vi "Main.vi"() -> ()   [LabVIEW 2015]
doc: "This Continuous Measurement sample project is based on the Queued Message Handler template.\n\nThe Event Handling Loop generates messages based on user interface actions.\n\nThe Message Handling Loop processes messages generated by the Event Handling Loop, or by other messages. There are also Acquisition and Logging message handling loop subVIs, and a chart updating loop."
uses:
  controls/UI Data.ctl
  controls/UI State.ctl
  Acquisition/Generic data packet.ctl
  My Graphs/Gps Map Graph coordinates.ctl
  Settings/Settings.ctl
  Acquisition/Hardware Configuration.ctl
  Logging/Logging Configuration.ctl
  My Graphs/Gps Map Graph config.ctl
  My Graphs/Chart to Graph enum.ctl
  Telemetria_Rotterdam_API_v2/TypeDef/data_graph.ctl
  My Graphs/Gps Map Graph enum.ctl
  Support VIs/Message Queue/Enqueue Message (Single).vi
  Support VIs/Message Queue/Enqueue Message (Array).vi
  <vilib>/Utility/error.llb/Error Cluster From Error Code.vi
  <vilib>/ErrorRing/Error Ring.xnode
  Acquisition/Acquisition.lvlib
  Logging/Logging.lvlib
  Settings/Settings.lvlib
  Support VIs/User Event - Stop/User Event - Stop.lvlib
  Support VIs/Message Queue/Message Queue.lvlib
  My Graphs/My Graphs.lvlib
panel:
  out "RX":bool
  out "EM_RPM_top":u16 caption="EM RPM"
  out "ICE_RPM_top":u16 caption="ICE RPM"
  out "Battery_voltage_top":sgl caption="Battery voltage"
  in  "Disconnect":bool
  out "Status":string
  in  "Exit_top":bool caption="Exit"
  out "Strategy_top":u8 caption="Strategy"
  out "ElettricMotor_top":bool caption="Electric\nMotor"
  out "Electronics_top":bool caption="Electronics"
  out "Emergency_top":bool caption="Emergency"
  out "Humidity2_top":sgl caption="Humidity 2"
  out "Humidity1_top":sgl caption="Humidity 1"
  out "Temperature3_top":sgl caption="Temperature 3"
  out "Temperature2_top":sgl caption="Temperature 2"
  out "Temperature1_top":sgl caption="Temperature 1" format="%_2f"
  out "Speed_top":sgl caption="Speed" format="%_3g"
  out "Current_top":sgl caption="Current" format="%_3f"
  out "Voltage_top":sgl caption="Voltage" format="%_4f"
  in  "Connect":bool
  in  "Tab Control":T1(tab)
  out "TimeRT":string caption="Time"
  out "Humidity 2":sgl(slide) scale=0.0..100.0
  out "Humidity 1":sgl(slide) scale=0.0..100.0
  out "Current":sgl(knob) scale=0.0..10.0
  out "Voltage":sgl(knob) scale=0.0..50.0
  out "Temperature 3":sgl(slide) scale=0.0..100.0
  out "Temperature 2":sgl(slide) scale=0.0..100.0
  out "Temperature 1":sgl(slide) scale=0.0..100.0
  out "Speed":sgl(knob) scale=0.0..40.0
  out "Map":cluster{"X":dbl, "Y":dbl}[](graph)
  out "Electric Motor RPM":u16(knob) scale=0.0..10000.0
  out "ICE RPM":u16(knob) scale=0.0..10000.0
  out "Battery voltage":sgl(knob) scale=0.0..50.0
  out "TimeM":string caption="Time"
  out "Mini Map":cluster{"X":dbl, "Y":dbl}[](graph)
  out "Voltage_Graph":cluster{"Tempi":dbl[], "Valori":dbl[]}[](graph) caption="Voltage"
  out "Current_Graph":cluster{"Tempi":dbl[], "Valori":dbl[]}[](graph) caption="Current"
  out "Speed_Graph":cluster{"Tempi":dbl[], "Valori":dbl[]}[](graph) caption="Speed"
  out "Humidities":cluster{"Tempi":dbl[], "Valori":dbl[]}[](graph) caption="Humidity"
  out "Temperatures":cluster{"Tempi":dbl[], "Valori":dbl[]}[](graph) caption="Temperature"
  out "Messages with wrong length":u32
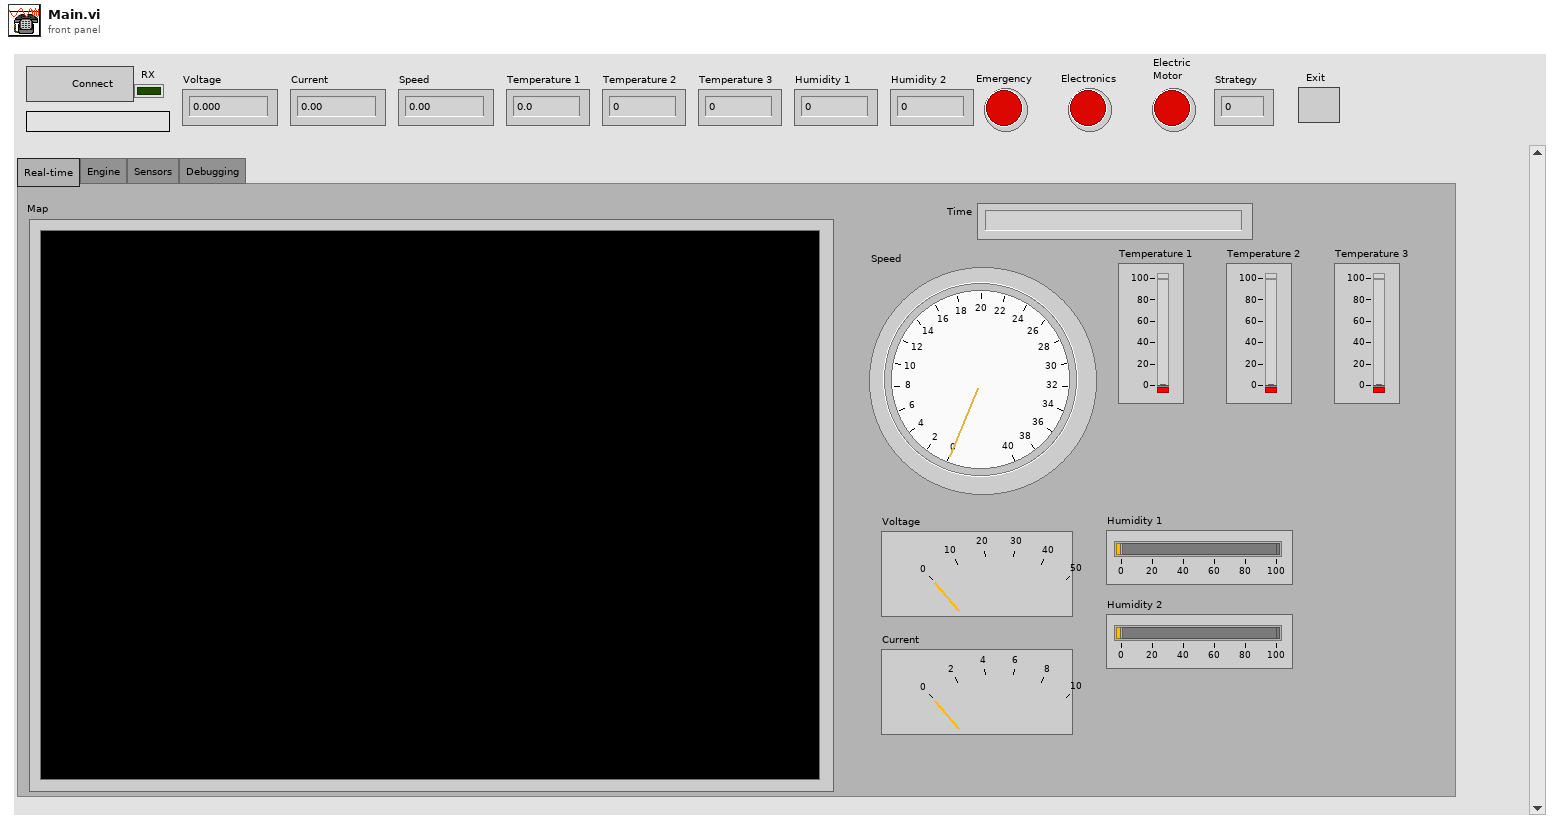
[diagram p1: front panel]
types:
  T1 = enum32{"Real-time", "Engine", "Sensors", "Debugging"}
  T2 = typedef "Settings.lvlib/Settings.ctl" = cluster{"Connection Configuration":T3, "Logging Configuration":T4, "Maps config":cluster{"Real-time map config":T5, "Mini map config":T5}, "Data format":enum16{"IDRA data", "XAM data"}}
  T3 = typedef "Acquisition.lvlib/Hardware Configuration.ctl" = cluster{"Data source":enum16{"Serial port", "Simulated data", "Web page JSON"}, "Connection info":cluster{"VISA resource name":refnum<visa-resource-name>, "Baud rate":u32, "data bits":u16, "stop bits":u16, "parity (0:none)":enum16{"None", "Odd", "Even", "Mark", "Space"}, "flow control (0:none)":u16, "timeout (10sec)":u32, "termination char\n(0xA = '\\n' = LF) ":u8, "Enable Termination\nChar (T)":bool}, "Protocol info":cluster{"Temination char":u8, "Escape char":u8}, "Internet server":cluster{"Web page telemetry":string, "Web page gps":string}, "Data format":enum16{"IDRA data", "XAM data"}}
  T4 = typedef "Logging.lvlib/Logging Configuration.ctl" = cluster{"Log File Base Path":path, "TDMS File Reference":refnum<k34>, "Data format":enum16{"IDRA data", "XAM data"}}
  T5 = typedef "Gps Map Graph config.ctl" = cluster{"Config path":path, "Image path":path}
  T6 = typedef "Acquisition.lvlib/Generic data packet.ctl" = cluster{"Content type":enum16{"None", "Telemetria", "GPS"}, "GPS":T7, "Telemetria":cluster{"Data format":enum16{"IDRA data", "XAM data"}, "Data":variant}}
  T7 = typedef "Gps Map Graph coordinates.ctl" = cluster{"Latitude":dbl, "Longitude":dbl}
  T8 = typedef "UI State.ctl" = enum16{"Idle", "Acquiring and Logging", "Waiting for Exit", "Waiting for Exit (Acq Stopped)", "Waiting for Exit (Log Stopped)", "Waiting for Stop", "Waiting for Stop (Acq Stopped)", "Waiting for Stop (Log Stopped)"}
  T9 = typedef "UI Data.ctl" = cluster{"Connect Ref":refnum<vi>, "Disconnect Ref":refnum<vi>, "Exit Ref":refnum<vi>, "Status Ref":refnum<vi>}
  T10 = typedef "Message Queue.lvlib/All Message Queues.ctl" = cluster{"UI":refnum<queue>, "Acquisition":refnum<queue>, "Logging":refnum<queue>}
  T11 = typedef "My Graphs.lvlib/Chart to Graph enum.ctl" = enum16{"AddValue", "Reset", "Delete_old"}
  T12 = typedef "My Graphs.lvlib/Gps Map Graph enum.ctl" = enum16{"Reset_ini", "Reset_txt", "SetValue"}
  T13 = cluster{"Real-time map config":T5, "Mini map config":T5}
  T14 = typedef "data_graph.ctl" = cluster{"Time":sgl, "Voltage":sgl, "Current":sgl, " Speed":sgl, "ID trasmitter":u8}
  T15 = typedef "Acquisition.lvlib/XAM Data Packet.ctl" = cluster{"Minutes":u16, "Seconds/100":u16, "Supercap Voltage":sgl, "Battery Voltage":sgl, "Supercap Current":sgl, "Speed":sgl, "EM Temperature":sgl, "ECU Temperature":sgl, "ICE Temperature":sgl, "RPM EM":u16, "RPM ICE":u16, "Cruise Control":bool, "Emergency":bool}
  T16 = typedef "Acquisition.lvlib/IDRA Data Packet.ctl" = cluster{"Minutes":u16, "Seconds/100":u16, "Voltage":sgl, "Current":sgl, "Speed":sgl, "Temperature 1":sgl, "Temperature 2":sgl, "Temperature 3":sgl, "Humidity 1":sgl, "Humidity 2":sgl, "Strategy":u8, "Electric Motor":bool, "Electronics":bool, "Emergency":bool}
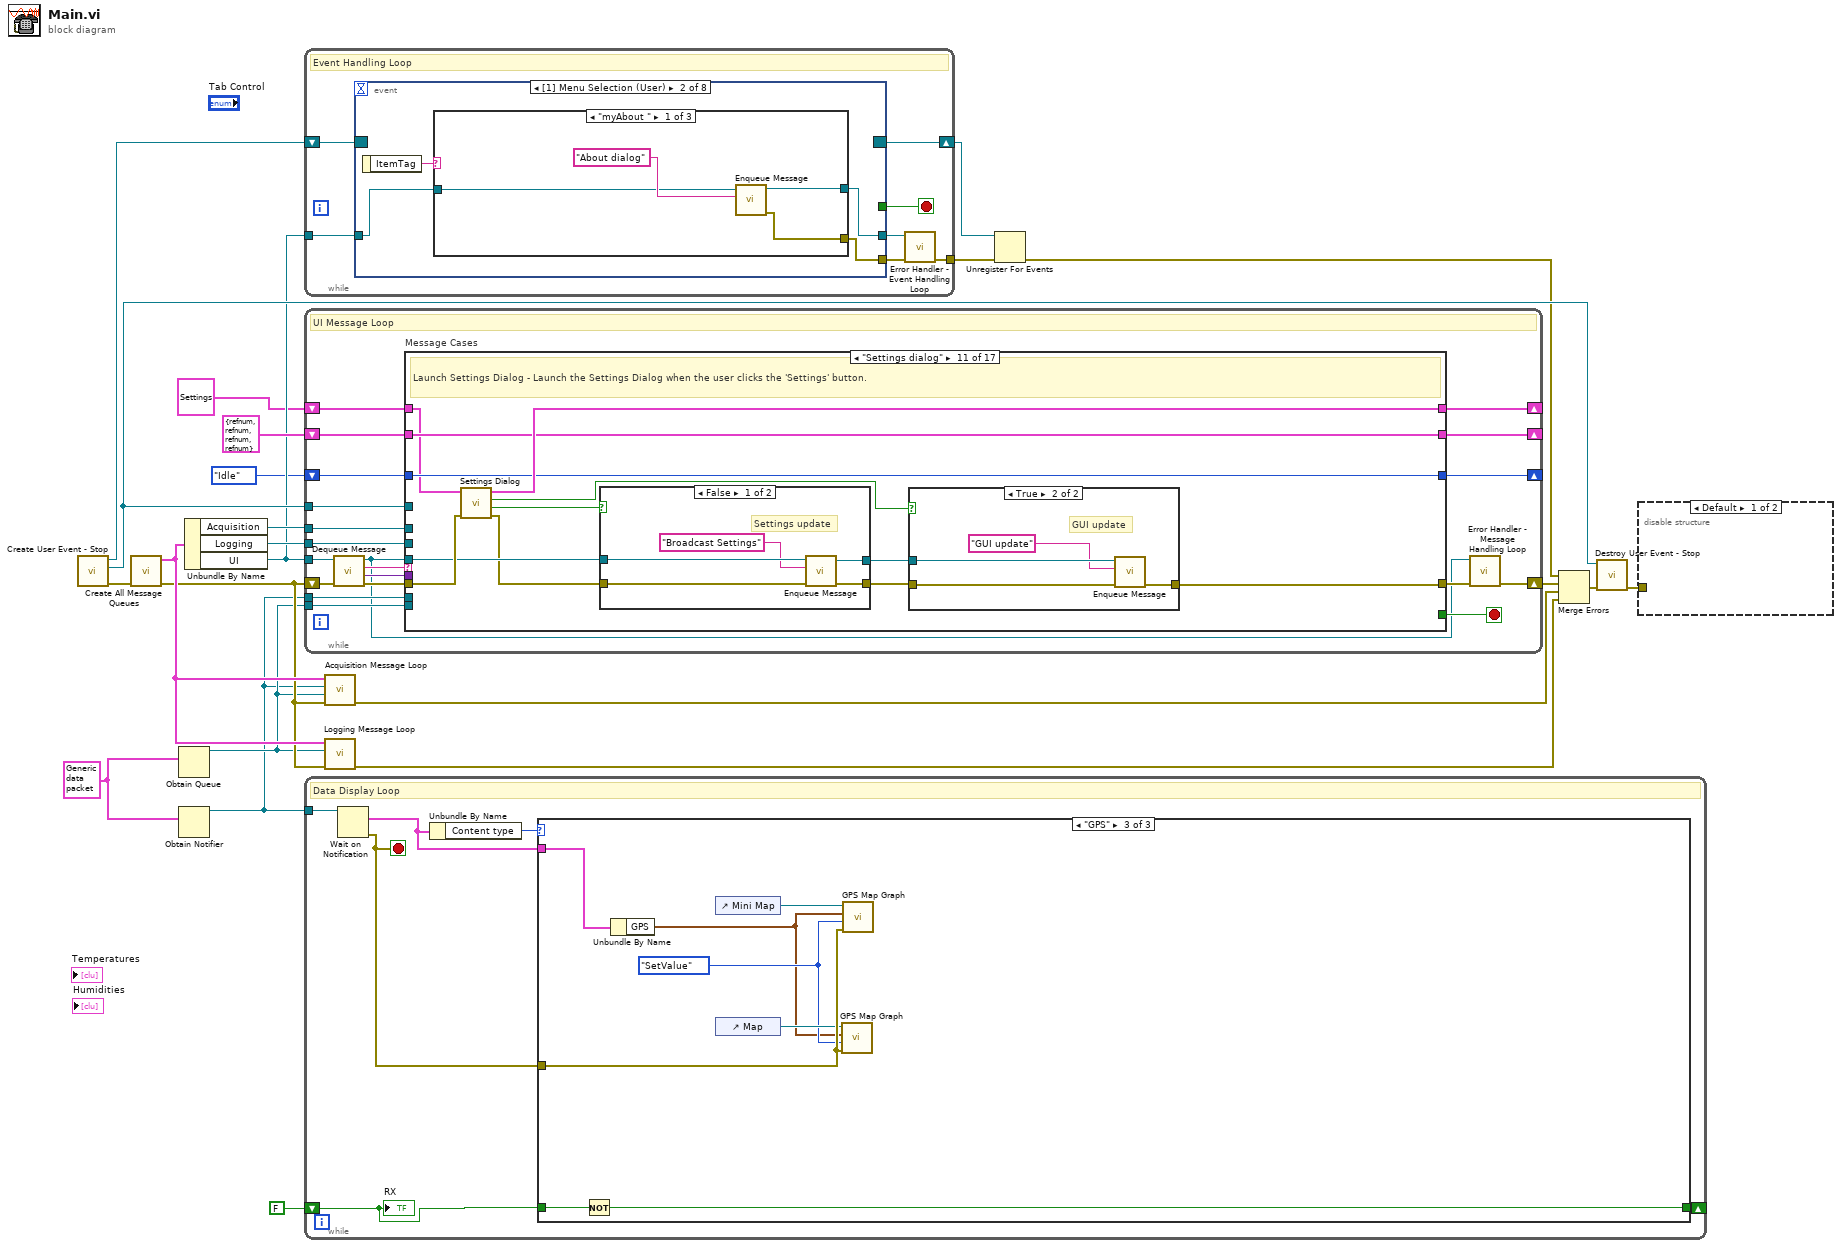
[diagram p0: block diagram]
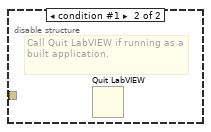
[diagram p2: hidden frame]
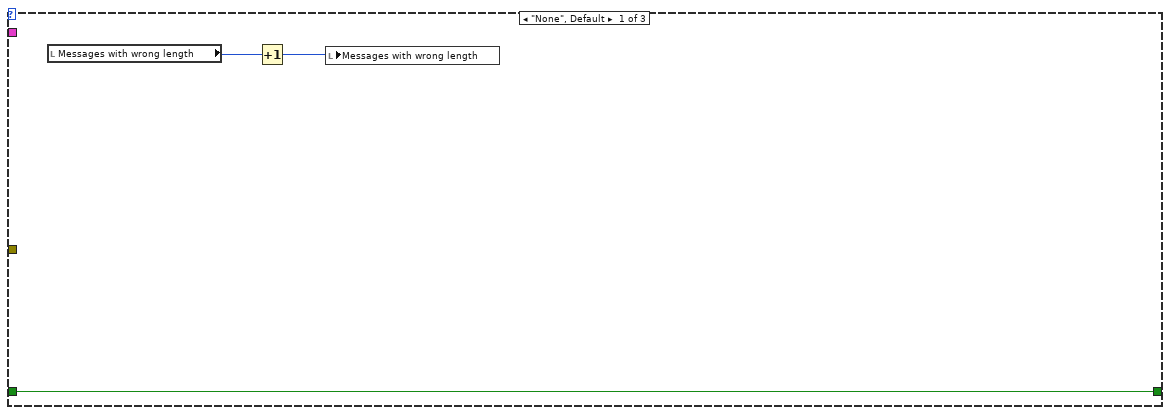
[diagram p3: hidden frame]
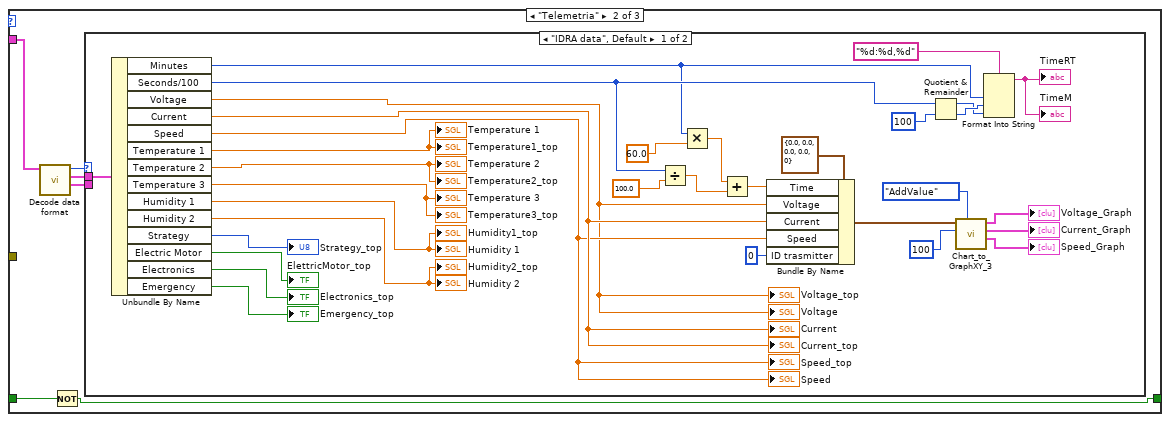
[diagram p4: hidden frame]
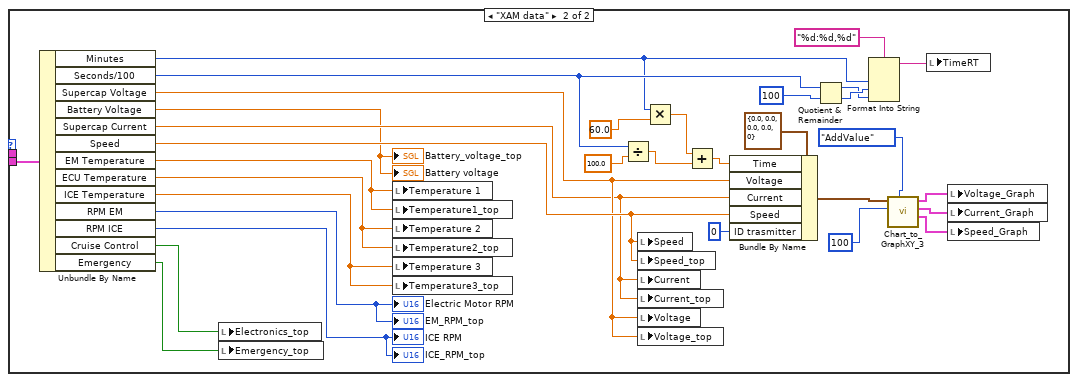
[diagram p5: hidden frame]
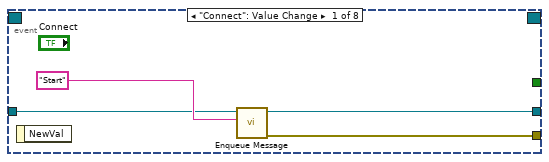
[diagram p6: hidden frame]
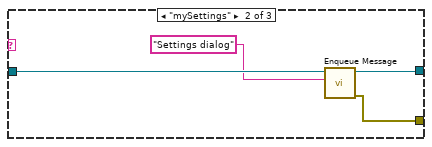
[diagram p7: hidden frame]
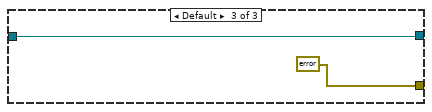
[diagram p8: hidden frame]
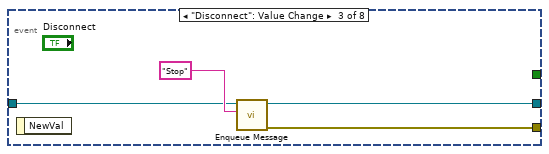
[diagram p9: hidden frame]
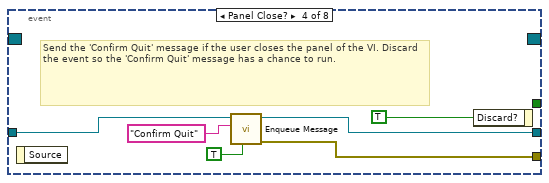
[diagram p10: hidden frame]
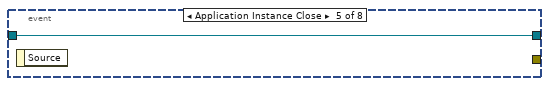
[diagram p11: hidden frame]
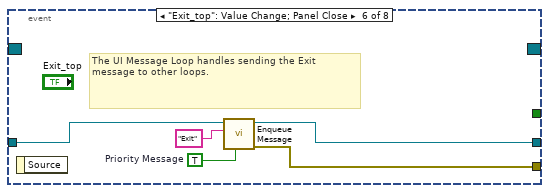
[diagram p12: hidden frame]
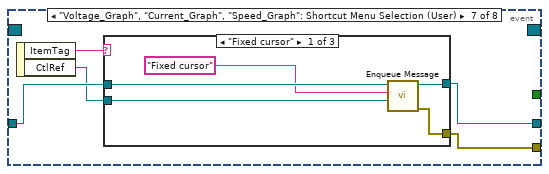
[diagram p13: hidden frame]
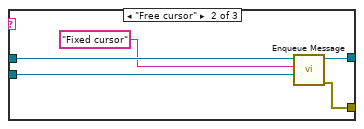
[diagram p14: hidden frame]
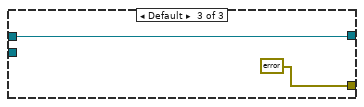
[diagram p15: hidden frame]
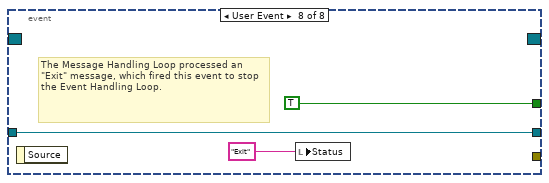
[diagram p16: hidden frame]
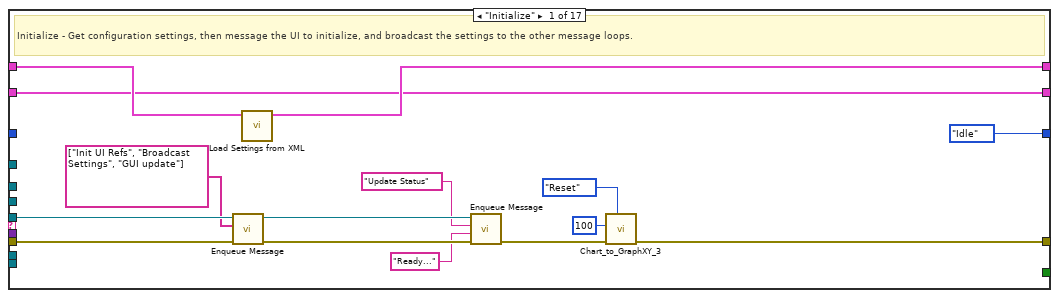
[diagram p17: hidden frame]
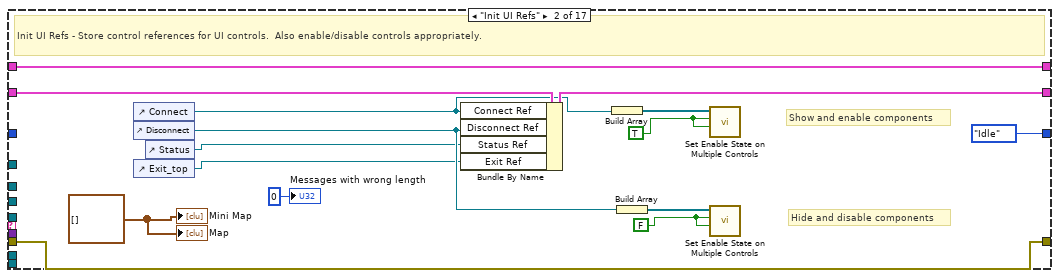
[diagram p18: hidden frame]
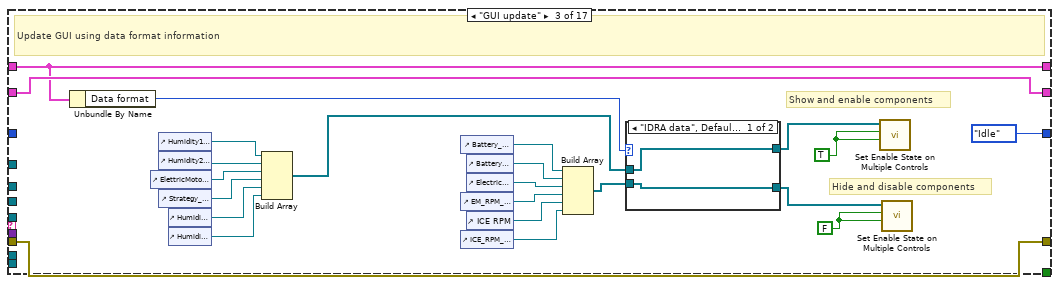
[diagram p19: hidden frame]
diagram:
  w3 = T6 {"Content type"=enum."None", "GPS"={"Latitude"=0.0, "Longitude"=0.0}, "Telemetria"={"Data format"=enum."IDRA data", "Data"=variant}}
  n1 = call "Create User Event - Stop.vi"() -> ("error out"=w18:errorcluster, "User Event - Stop"=w20:refnum<user-event>, "Stop Event Registration Refnum"=w21:refnum<event-registration>)  [unwired: 9 in]
  n2 = call "Create All Message Queues.vi"("error in (no error)"=w18) -> ("error out"=w15:errorcluster, "Message Queues out"=w17:T10)  [unwired: 9 in]
  n3 = Obtain Queue(element data type=w3) -> (queue out=w8:refnum<queue>)  [unwired: 4 in, 2 out]
  n4 = Obtain Notifier(notification data type=w3) -> (notifier out=w4:refnum<notifier>)  [unwired: 3 in, 2 out]
  n5 = Unbundle By Name(w17) -> ("Acquisition"=w11:refnum<queue>, "Logging"=w10:refnum<queue>, "UI"=w9:refnum<queue>)
  n6 = while {
    tunnel: w9 -> [w29]
    tunnel: [w26] -> w22
    shift-right: [w28] -> w13
    shift-left: w21 -> [w30]
    stop <- w27 stop-if-true
    # "Event Handling Loop"
    n7 = event shown="[1] Menu Selection (User)" {
      selector: w30 -> [_ _ _ _ _ _ _ _]
      dyn-events: [_ _ _ _ _ _ _ _] -> w28
      timeout: _ -> [_ _ _ _ _ _ _ _]
      tunnel: [_ _ _ _ _ _ _ TRUE ("Discard?")] -> w27
      tunnel: w29 -> [w32 w37 w51 w56 w59 w61 w68 w82]
      tunnel: [w34 w35 w50 w54 _ w64 w66 _] -> w25
      tunnel: [w31 w36 w49 w55 w59 w60 w67 w82] -> w24
      event "Connect": Value Change {
        n8 = event-data() -> ()  [unwired: 1 in, 1 out]
        n9 = call-poly "Enqueue Message.vi"("Message"="Start", "Message Queue"=w32) -> ("error out"=w34:errorcluster, "dup Message Queue"=w31:refnum<queue>)  [unwired: 8 in]
      }
      event Menu Selection (User) {
        n10 = event-data() -> ("ItemTag"=w38:string)  [unwired: 1 in]
        n11 = case shown="\"myAbout \"" w38 {
          tunnel: w37 -> [w41 w46 w48]
          tunnel: [w40 w45 w48] -> w36
          tunnel: [w39 w44 errorcluster {"status"=FALSE, "code"=0, "source"=""} ("error out")] -> w35
          frame "myAbout " {
            n12 = call-poly "Enqueue Message.vi"("Message"="About dialog", "Message Queue"=w41) -> ("error out"=w39:errorcluster, "dup Message Queue"=w40:refnum<queue>)  [unwired: 8 in]
          }
          frame "mySettings" {
            n13 = call-poly "Enqueue Message.vi"("Message"="Settings dialog", "Message Queue"=w46) -> ("error out"=w44:errorcluster, "dup Message Queue"=w45:refnum<queue>)  [unwired: 8 in]
          }
          frame Default {
          }
        }
      }
      event "Disconnect": Value Change {
        n14 = event-data() -> ()  [unwired: 1 in, 1 out]
        n15 = call-poly "Enqueue Message.vi"("Message"="Stop", "Message Queue"=w51) -> ("error out"=w50:errorcluster, "dup Message Queue"=w49:refnum<queue>)  [unwired: 8 in]
      }
      event Panel Close? {
        # "Send the 'Confirm Quit' message if the user closes the panel of the VI. Discard the event so the 'Confirm Quit' message has a chance to run."
        n16 = event-data() -> ()  [unwired: 1 in, 1 out]
        n17 = call-poly "Enqueue Message.vi"("Priority Message? (F)"=TRUE, "Message"="Confirm Quit", "Message Queue"=w56) -> ("error out"=w54:errorcluster, "dup Message Queue"=w55:refnum<queue>)  [unwired: 7 in]
        n18 = event-data("Discard?"=TRUE) -> ()  [unwired: 1 in, 1 out]
      }
      event Application Instance Close {
        n19 = event-data() -> ()  [unwired: 1 in, 1 out]
      }
      event "Exit_top": Value Change; Panel Close {
        w62 = TRUE  # Priority Message
        # "The UI Message Loop handles sending the Exit message to other loops."
        n20 = event-data() -> ()  [unwired: 1 in, 1 out]
        n21 = call-poly "Enqueue Message.vi"("Priority Message? (F)"=w62, "Message"="Exit", "Message Queue"=w61) -> ("error out"=w64:errorcluster, "dup Message Queue"=w60:refnum<queue>)  [unwired: 7 in]
      }
      event "Voltage_Graph", "Current_Graph", "Speed_Graph": Shortcut Menu Selection (User) {
        n22 = event-data() -> ("ItemTag"=w69:string, "CtlRef"=w65:refnum<vi>)  [unwired: 1 in]
        n23 = case shown="\"Fixed cursor\"" w69 {
          tunnel: w68 -> [w73 w79 w81]
          tunnel: [w74 w78 w81] -> w67
          tunnel: [w72 w77 errorcluster {"status"=FALSE, "code"=0, "source"=""} ("error out")] -> w66
          tunnel: w65 -> [w70 w75 _]
          frame "Fixed cursor" {
            n24 = call-poly "Enqueue Message.vi"("Message Data"=w70, "Message"="Fixed cursor", "Message Queue"=w73) -> ("error out"=w72:errorcluster, "dup Message Queue"=w74:refnum<queue>)  [unwired: 7 in]
          }
          frame "Free cursor" {
            n25 = call-poly "Enqueue Message.vi"("Message Data"=w75, "Message"="Fixed cursor", "Message Queue"=w79) -> ("error out"=w77:errorcluster, "dup Message Queue"=w78:refnum<queue>)  [unwired: 7 in]
          }
          frame Default {
          }
        }
      }
      event User Event {
        # "The Message Handling Loop processed an \"Exit\" message, which fired this event to stop the Event Handling Loop."
        n26 = event-data() -> ()  [unwired: 1 in, 1 out]
        n27 = local write "Status"("Exit" ("Exit String")) -> ()
      }
    }
    n28 = call "Error Handler - Event Handling Loop.vi"("error in (no error)"=w25, "Message Queue"=w24) -> ("dup error in"=w26:errorcluster)  [unwired: 8 in, 1 out]
  }
  n29 = while {
    tunnel: w9 -> [w98]
    tunnel: w20 -> [w103]
    shift-right: [w89] -> w23
    shift-left: w15 -> [w102]
    shift-right: [w97] -> _
    shift-left: T2 {"Connection Configuration"={"Data source"=enum."Serial port", "Connection info"={"VISA resource name"="COM 1", "Baud rate"=9600, "data bits"=8, "stop bits"=0, "parity (0:none)"=enum."None", "flow control (0:none)"=0, "timeout (10sec)"=10000, "termination char\n(0xA = '\\n' = LF) "=10, "Enable Termination\nChar (T)"=TRUE}, "Protocol info"={"Temination char"=255, "Escape char"=254}, "Internet server"={"Web page telemetry"="", "Web page gps"=""}, "Data format"=enum."IDRA data"}, "Logging Configuration"={"Log File Base Path"=path "", "TDMS File Reference"=refnum, "Data format"=enum."IDRA data"}, "Maps config"={"Real-time map config"={"Config path"=path "", "Image path"=path ""}, "Mini map config"={"Config path"=path "", "Image path"=path ""}}, "Data format"=enum."IDRA data"} ("Settings in") -> [w96]
    shift-right: [w94] -> _
    shift-left: T9 {"Connect Ref"=refnum, "Disconnect Ref"=refnum, "Exit Ref"=refnum, "Status Ref"=refnum} ("Measurement UI Controls") -> [w95]
    tunnel: w11 -> [w93]
    tunnel: w10 -> [w92]
    tunnel: w4 -> [w91]
    tunnel: w8 -> [w90]
    shift-right: [w85] -> _
    shift-left: UI_State."Idle" ("UI State") -> [w86]
    stop <- w104 stop-if-true
    # "UI Message Loop"
    n30 = call "Dequeue Message.vi"("error in (no error)"=w102, "Message Queue"=w98) -> ("error out"=w101:errorcluster, "Message Data"=w99:variant, "Message"=w100:string, "dup Message Queue"=w87:refnum<queue>)  [unwired: 6 in]
    n31 = case "Message Cases" shown="\"Settings dialog\"" w100 {
      selector: w100 -> [_ _ _ _ _ _ _ _ _ _ _ _ _ _ _ _ w382]
      tunnel: w87 -> [w112 _ _ _ _ w198 _ w221 w246 _ w299 w318 w329 w360 _ _ _]
      tunnel: w101 -> [w111 w120 w152 w169 w172 w197 w215 w222 w247 w283 w300 w321 w328 w368 w375 w380 _]
      tunnel: [w107 w120 w152 w170 w176 w184 w216 w219 w244 w288 w292 w317 w327 w369 w374 w379 w381] -> w88
      tunnel: [_ _ _ _ _ _ _ _ _ _ _ _ _ TRUE _ _ _] -> w104
      tunnel: w99 -> [_ _ _ w168 _ _ _ _ _ _ _ w319 _ _ _ _ _]
      tunnel: w103 -> [_ _ _ _ _ _ _ _ _ _ _ _ _ w367 _ _ _]
      tunnel: [w118 w134 w153 w164 w175 w196 w214 w225 w250 w286 w298 w325 w332 w365 w373 w378 w385] -> w97
      tunnel: w96 -> [w119 w134 w153 w164 w175 w196 w214 w225 w250 w286 w289 w325 w332 w365 w373 w378 w385]
      tunnel: w95 -> [w113 w133 w154 w163 w174 w193 w213 w224 w249 w281 w296 w324 w331 w363 w372 w377 w384]
      tunnel: [w113 w132 w154 w163 w174 w193 w213 w224 w249 w281 w296 w324 w331 w363 w372 w377 w384] -> w94
      tunnel: w93 -> [_ _ _ _ _ w183 w204 _ _ w280 _ _ _ w362 _ _ _]
      tunnel: w92 -> [_ _ _ _ _ w186 w207 _ _ w279 _ _ _ w361 _ _ _]
      tunnel: w91 -> [_ _ _ _ _ _ _ _ _ _ _ _ _ w359 _ _ _]
      tunnel: w90 -> [_ _ _ _ _ _ _ _ _ _ _ _ _ w355 _ _ _]
      tunnel: w86 -> [_ _ _ w162 w173 _ w201 w223 w248 w278 w295 w313 w330 _ w371 w376 w383]
      tunnel: [UI_State."Idle" ("UI State") UI_State."Idle" ("UI State") UI_State."Idle" ("UI State") w162 w173 UI_State."Acquiring and Logging" ("UI State") w202 w220 w245 w278 w295 w313 w326 UI_State."Idle" ("UI State") w371 w376 w383] -> w85
      frame "Initialize" {
        # "Initialize - Get configuration settings, then message the UI to initialize, and broadcast the settings to the other message loops."
        n32 = call-poly "Enqueue Message.vi"("error in (no error)"=w111, "Message Array"=string[] ["Init UI Refs", "Broadcast Settings", "GUI update"], "Message Queue"=w112) -> ("error out"=w117:errorcluster, "dup Message Queue"=w116:refnum<queue>)  [unwired: 7 in]
        n33 = call "Load Settings from XML.vi"("Settings in"=w119) -> ("Settings out"=w118:T2)  [unwired: 9 in, 1 out]
        n34 = call-poly "Enqueue Message.vi"("error in (no error)"=w117, "Message Data"="Ready..." ("Ready..."), "Message"="Update Status", "Message Queue"=w116) -> ("error out"=w108:errorcluster)  [unwired: 6 in, 1 out]
        n35 = call "Chart_to_GraphXY_3.vi"("Function"=Chart_to_Graph_enum."Reset", "Error In"=w108, "Time window"=100) -> ("Error Out"=w107:errorcluster)  [unwired: 5 in, 3 out]
      }
      frame "Init UI Refs" {
        w121 = cluster{"X":dbl, "Y":dbl}[] [] ("Mini Map")
        w123 = FALSE ("Enable?")
        w124 = TRUE ("Enable?")
        # "Hide and disable components"
        # "Show and enable components"
        # "Init UI Refs - Store control references for UI controls.  Also enable/disable controls appropriately."
        n36 = control-ref of="Connect"() -> (w125:refnum<vi>)
        n37 = control-ref of="Disconnect"() -> (w129:refnum<vi>)
        n38 = control-ref of="Exit_top"() -> (w128:refnum<vi>)
        n39 = control-ref of="Status"() -> (w126:refnum<vi>)
        n40 = Bundle By Name(cluster=w133, "Connect Ref"=w125, "Disconnect Ref"=w129, "Status Ref"=w126, "Exit Ref"=w128) -> (w132:T9)
        n41 = Build Array(w125) -> (w131:refnum<vi>[])
        n42 = Build Array(w129) -> (w130:refnum<vi>[])
        n43 = call "Set Enable State on Multiple Controls.vi"("Visible?"=w124, "Enable?"=w124, "Controls"=w131) -> ()  [unwired: 9 in]
        n44 = call "Set Enable State on Multiple Controls.vi"("Visible?"=w123, "Enable?"=w123, "Controls"=w130) -> ()  [unwired: 9 in]
        "Messages with wrong length" <- u32 0 ("Messages with wrong length")
        "Mini Map" <- w121
        "Map" <- w121
      }
      frame "GUI update" {
        w155 = FALSE ("Enable?")
        w156 = TRUE ("Enable?")
        # "Hide and disable components"
        # "Show and enable components"
        # "Update GUI using data format information"
        n45 = Unbundle By Name(w153) -> ("Data format"=w139:enum16{"IDRA data", "XAM data"})
        n46 = control-ref of="ElettricMotor_top"() -> (w149:refnum<vi>)
        n47 = control-ref of="Humidity1_top"() -> (w151:refnum<vi>)
        n48 = control-ref of="Humidity2_top"() -> (w150:refnum<vi>)
        n49 = control-ref of="Strategy_top"() -> (w148:refnum<vi>)
        n50 = control-ref of="Humidity 1"() -> (w147:refnum<vi>)
        n51 = control-ref of="Humidity 2"() -> (w146:refnum<vi>)
        n52 = Build Array(w151, w150, w149, w148, w147, w146) -> (w138:refnum<vi>[])
        n53 = control-ref of="Battery_voltage_top"() -> (w145:refnum<vi>)
        n54 = control-ref of="EM_RPM_top"() -> (w142:refnum<vi>)
        n55 = control-ref of="ICE_RPM_top"() -> (w140:refnum<vi>)
        n56 = control-ref of="Battery voltage"() -> (w144:refnum<vi>)
        n57 = control-ref of="Electric Motor RPM"() -> (w143:refnum<vi>)
        n58 = control-ref of="ICE RPM"() -> (w141:refnum<vi>)
        n59 = Build Array(w145, w144, w143, w142, w141, w140) -> (w137:refnum<vi>[])
        n60 = case shown="\"IDRA data\", Default" w139 {
          tunnel: w138 -> [w159 w160]
          tunnel: w137 -> [w158 w161]
          tunnel: [w159 w161] -> w136
          tunnel: [w158 w160] -> w135
          frame "IDRA data", Default {
          }
          frame "XAM data" {
          }
        }
        n61 = call "Set Enable State on Multiple Controls.vi"("Visible?"=w156, "Enable?"=w156, "Controls"=w136) -> ()  [unwired: 9 in]
        n62 = call "Set Enable State on Multiple Controls.vi"("Visible?"=w155, "Enable?"=w155, "Controls"=w135) -> ()  [unwired: 9 in]
      }
      frame "Update Status" {
        # "barra di stato corrente"
        # "Update Display - Convert the message data to a string to display in the Status indicator."
        n63 = Variant To Data(error in=w169, type="", Variant=w168) -> (data=→"Status":string, error out=w166:errorcluster)
        n64 = Merge Errors(w166) -> (w170:errorcluster)
      }
      frame "About dialog" {
        # "Update Display - Convert the message data to a string to display in the Status indicator."
        n65 = flat-sequence {
          tunnel: w172 -> [w178]
          tunnel: [w178] -> w171
          frame #0 {
            n66 = One Button Dialog(message="Telemetria H2politO\nv 0.3 - 2014\nRealizzatori:\nFausto Annicchiarico Petruzzelli\nMarco Lucarella") -> ()  [unwired: 1 in, 1 out]
          }
        }
        n67 = Merge Errors(w171) -> (w176:errorcluster)
      }
      frame "Start" {
        w180 = FALSE ("Enable?")
        w179 = TRUE ("Enable?")
        # "Message Acquisition and Logging loops to start."
        # "Start - Enable/Disable buttons appropriately for an acquisition that has started, and update status display."
        n68 = Unbundle By Name(w193) -> ("Connect Ref"=w190:refnum<vi>, "Disconnect Ref"=w189:refnum<vi>)
        n69 = call-poly "Enqueue Message.vi"("error in (no error)"=w197, "Message Data"="Acquiring and Logging..." ("Acquiring and Logging..."), "Message"="Update Status", "Message Queue"=w198) -> ("error out"=w188:errorcluster)  [unwired: 6 in, 1 out]
        n70 = Build Array(w189) -> (w192:refnum<vi>[])
        n71 = Build Array(w190) -> (w191:refnum<vi>[])
        n72 = call "Set Enable State on Multiple Controls.vi"("Visible?"=w180, "Enable?"=w180, "Controls"=w191) -> ()  [unwired: 9 in]
        n73 = call "Set Enable State on Multiple Controls.vi"("Visible?"=w179, "Enable?"=w179, "Controls"=w192) -> ()  [unwired: 9 in]
        n74 = call-poly "Enqueue Message.vi"("error in (no error)"=w188, "Message"="Start", "Message Queue"=w186) -> ("error out"=w185:errorcluster)  [unwired: 7 in, 1 out]
        n75 = call-poly "Enqueue Message.vi"("error in (no error)"=w185, "Message"="Start", "Message Queue"=w183) -> ("error out"=w184:errorcluster)  [unwired: 7 in, 1 out]
      }
      frame "Stop" {
        w199 = TRUE ("Enable?")
        w200 = FALSE ("Enable?")
        # "Message Acquisition and Logging loops to stop"
        # "Stop - Enable/Disable buttons appropriately for an acquisition that has stopped, and update status display."
        n76 = Unbundle By Name(w213) -> ("Connect Ref"=w210:refnum<vi>, "Disconnect Ref"=w209:refnum<vi>)
        n77 = Build Array(w209) -> (w212:refnum<vi>[])
        n78 = Build Array(w210) -> (w211:refnum<vi>[])
        n79 = call "Set Enable State on Multiple Controls.vi"("Visible?"=w199, "Enable?"=w199, "Controls"=w211) -> ()  [unwired: 9 in]
        n80 = call "Set Enable State on Multiple Controls.vi"("Visible?"=w200, "Enable?"=w200, "Controls"=w212) -> ()  [unwired: 9 in]
        n81 = call-poly "Enqueue Message.vi"("error in (no error)"=w215, "Message"="Stop", "Message Queue"=w207) -> ("error out"=w206:errorcluster)  [unwired: 7 in, 1 out]
        n82 = case shown="Default" w201 {
          selector: w201 -> [w217 _]
          tunnel: [w217 UI_State."Waiting for Stop" ("UI State")] -> w202
          frame "Waiting for Exit" {
          }
          frame Default {
          }
        }
        n83 = call-poly "Enqueue Message.vi"("error in (no error)"=w206, "Message"="Stop", "Message Queue"=w204) -> ("error out"=w205:errorcluster)  [unwired: 7 in, 1 out]
        n84 = Merge Errors(w205) -> (w216:errorcluster)
      }
      frame "Acquisition Stopped" {
        # "Logic for determining what action to take when the acquisition has stopped."
        n85 = case shown="\"Waiting for Exit (Log Stopped)\"" w223 {
          selector: w223 -> [w227 _ _ _ _]
          tunnel: w222 -> [w226 w229 w231 w237 w243]
          tunnel: w221 -> [_ _ _ w235 w240]
          tunnel: [w227 UI_State."Waiting for Exit (Acq Stopped)" ("UI State") UI_State."Waiting for Stop (Acq Stopped)" ("UI State") UI_State."Idle" ("UI State") UI_State."Idle" ("UI State")] -> w220
          tunnel: [w226 w229 w231 w236 w241] -> w219
          frame Default {
          }
          frame "Waiting for Exit", "Waiting for Exit (Acq Stopped)" {
          }
          frame "Waiting for Stop", "Waiting for Stop (Acq Stopped)" {
          }
          frame "Waiting for Exit (Log Stopped)" {
            # "If we are waiting to exit, and the logging has already stopped, then the \"Acquisition Stopped\" message indicates that it is time to exit."
            n86 = call-poly "Enqueue Message.vi"("Priority Message? (F)"=TRUE, "error in (no error)"=w237, "Message"="Exit", "Message Queue"=w235) -> ("error out"=w236:errorcluster)  [unwired: 6 in, 1 out]
          }
          frame "Waiting for Stop (Log Stopped)" {
            # "If we are waiting to stop, and the logging has already stopped, then the \"Acquisition Stopped\" message indicates that it is time to stop."
            n87 = call-poly "Enqueue Message.vi"("error in (no error)"=w243, "Message Data"="Ready..." ("Ready..."), "Message"="Update Status", "Message Queue"=w240) -> ("error out"=w241:errorcluster)  [unwired: 6 in, 1 out]
          }
        }
      }
      frame "Logging Stopped" {
        # "Logic for determining what action to take when the logging has stopped."
        n88 = case shown="\"Waiting for Stop (Acq Stopped)\"" w248 {
          selector: w248 -> [w252 _ _ _ _]
          tunnel: w247 -> [w251 w254 w256 w262 w265]
          tunnel: w246 -> [_ _ _ w260 w264]
          tunnel: [w252 UI_State."Waiting for Exit (Log Stopped)" ("UI State") UI_State."Waiting for Stop (Log Stopped)" ("UI State") UI_State."Idle" ("UI State") UI_State."Idle" ("UI State")] -> w245
          tunnel: [w251 w254 w256 w261 w263] -> w244
          frame Default {
          }
          frame "Waiting for Exit", "Waiting for Exit (Log Stopped)" {
          }
          frame "Waiting for Stop", "Waiting for Stop (Log Stopped)" {
          }
          frame "Waiting for Exit (Acq Stopped)" {
            # "If we are waiting to exit, and the acquisition has already stopped, then the \"Logging Stopped\" message indicates that it is time to exit."
            n89 = call-poly "Enqueue Message.vi"("Priority Message? (F)"=TRUE, "error in (no error)"=w262, "Message"="Exit", "Message Queue"=w260) -> ("error out"=w261:errorcluster)  [unwired: 6 in, 1 out]
          }
          frame "Waiting for Stop (Acq Stopped)" {
            # "If we are waiting to stop, and the acquisition has already stopped, then the \"Logging Stopped\" message indicates that it is time to stop."
            n90 = call-poly "Enqueue Message.vi"("error in (no error)"=w265, "Message Data"="Ready..." ("Ready..."), "Message"="Update Status", "Message Queue"=w264) -> ("error out"=w263:errorcluster)  [unwired: 6 in, 1 out]
          }
        }
      }
      frame "Broadcast settings" {
        w274 = Gps_Map_Graph_enum."Reset_txt" ("Function")
        w282 = "Update Settings" ("Message")
        # "Broadcast settings - Send the 'Update Settings' message to the Logging and Acquisition message loops."
        n91 = Unbundle By Name(w286) -> ("Connection Configuration"=w285:T3, "Logging Configuration"=w284:T4, "Maps config"=w269:T13)
        n92 = call-poly "Enqueue Message.vi"("Message Data"=w285, "Message"=w282, "Message Queue"=w280) -> ("error out"=w287:errorcluster)  [unwired: 7 in, 1 out]
        n93 = call-poly "Enqueue Message.vi"("error in (no error)"=w287, "Message Data"=w284, "Message"=w282, "Message Queue"=w279) -> ("error out"=w277:errorcluster)  [unwired: 6 in, 1 out]
        n94 = Unbundle By Name(w269) -> ("Real-time map config"=w273:T5, "Mini map config"=w272:T5)
        n95 = control-ref of="Mini Map"() -> (w271:refnum<vi>)
        n96 = control-ref of="Map"() -> (w270:refnum<vi>)
        n97 = call "GPS Map Graph.vi"("Map config"=w272, "Error In"=w277, "Function"=w274, "Map ref in"=w271) -> ("Error Out"=w276:errorcluster)  [unwired: 6 in, 1 out]
        n98 = call "GPS Map Graph.vi"("Map config"=w273, "Error In"=w276, "Function"=w274, "Map ref in"=w270) -> ("Error Out"=w275:errorcluster)  [unwired: 6 in, 1 out]
        n99 = Merge Errors(w275, w283) -> (w288:errorcluster)
      }
      frame "Settings dialog" {
        # "Launch Settings Dialog - Launch the Settings Dialog when the user clicks the 'Settings' button."
        n100 = call "Settings Dialog.vi"("error in (no error)"=w300, "Settings in"=w289) -> ("error out"=w297:errorcluster, "Cancelled?"=w294:bool, "UI Refresh Needed?"=w290:bool, "Settings out"=w298:T2)  [unwired: 6 in]
        n101 = case shown="False" w294 {
          tunnel: w299 -> [w310 w311]
          tunnel: w297 -> [w309 w312]
          tunnel: [w308 w312] -> w293
          tunnel: [w306 w311] -> w291
          frame False {
            # "Settings update"
            n102 = call-poly "Enqueue Message.vi"("error in (no error)"=w309, "Message"="Broadcast Settings", "Message Queue"=w310) -> ("error out"=w308:errorcluster, "dup Message Queue"=w306:refnum<queue>)  [unwired: 7 in]
          }
          frame True {
          }
        }
        n103 = case shown="True" w290 {
          tunnel: w291 -> [_ w305]
          tunnel: w293 -> [w301 w304]
          tunnel: [w301 w303] -> w292
          frame False {
          }
          frame True {
            # "GUI update"
            n104 = call-poly "Enqueue Message.vi"("error in (no error)"=w304, "Message"="GUI update", "Message Queue"=w305) -> ("error out"=w303:errorcluster)  [unwired: 7 in, 1 out]
          }
        }
      }
      frame "Error" {
        # "Error - Check the error message data and respond accordingly. This message is sent by the \"Error Handler\" VIs at the end of each loop in this application."
        n105 = Variant To Data(error in=w321, type=errorcluster {"status"=FALSE, "code"=0, "source"=""} ("error constant"), Variant=w319) -> (data=w323:errorcluster, error out=w320:errorcluster)
        n106 = call <vilib>:"Simple Error Handler.vi"("error in (no error)"=w323) -> ()  [unwired: 4 in, 5 out]
        n107 = call-poly "Enqueue Message.vi"("Priority Message? (F)"=TRUE, "Message"="Exit", "Message Queue"=w318) -> ("error out"=w316:errorcluster)  [unwired: 7 in, 1 out]
        n108 = Merge Errors(w316, w320) -> (w317:errorcluster)
      }
      frame "Confirm Quit" {
        # "Confirm Quit - Message that can confirm whether or not the user wants to exit the application."
        n109 = case shown="\"Acquiring and Logging\"" w330 {
          tunnel: w329 -> [w338 w342]
          tunnel: w328 -> [w337 w341]
          tunnel: [w336 w340] -> w327
          tunnel: [UI_State."Idle" ("UI State") w339] -> w326
          frame Default {
            # "If 'Confirm Quit' comes in while the system is idle, there is no need for a confirmation message."
            n110 = call-poly "Enqueue Message.vi"("Priority Message? (F)"=TRUE, "error in (no error)"=w337, "Message"="Exit", "Message Queue"=w338) -> ("error out"=w336:errorcluster)  [unwired: 6 in, 1 out]
          }
          frame "Acquiring and Logging" {
            n111 = Two Button Dialog(message="Are you sure you want to quit while the acquisition is running?" ("Confirm Quit Message"), 1:"No" ("No"), 2:"Yes" ("Yes")) -> (T button?=w343:bool)
            n112 = case shown="True" w343 {
              tunnel: w342 -> [_ w352]
              tunnel: w341 -> [w348 w353]
              tunnel: [w348 w351] -> w340
              tunnel: [UI_State."Acquiring and Logging" ("UI State") UI_State."Waiting for Exit" ("UI State")] -> w339
              frame False {
                # "User did not want to quit."
              }
              frame True {
                n113 = call-poly "Enqueue Message.vi"("error in (no error)"=w353, "Message"="Stop", "Message Queue"=w352) -> ("error out"=w351:errorcluster)  [unwired: 7 in, 1 out]
              }
            }
          }
        }
      }
      frame "Exit" {
        w364 = "Exit" ("Message")
        # "Don't check the error outs. The acquisition and logging queues may have already been released."
        # "Close references owned by the Main VI."
        # "Stop the VI"
        # "Exit - Fire the User Event to stop the Event Handling Loop.  Also send Exit messages to the Acquisition and Logging loops."
        n114 = Release Queue(queue=w360, error in (no error)=w368) -> (error out=w358:errorcluster)  [unwired: 1 in, 2 out]
        n115 = call "Fire User Event - Stop.vi"("User Event - Stop"=w367) -> ("error out"=w366:errorcluster)  [unwired: 10 in]
        n116 = Release Notifier(notifier=w359, error in (no error)=w358) -> (error out=w357:errorcluster)  [unwired: 1 in, 2 out]
        n117 = Release Queue(queue=w355, error in (no error)=w357) -> (error out=w356:errorcluster)  [unwired: 1 in, 2 out]
        n118 = call-poly "Enqueue Message.vi"("Message"=w364, "Message Queue"=w362) -> ()  [unwired: 8 in, 2 out]
        n119 = call-poly "Enqueue Message.vi"("Message"=w364, "Message Queue"=w361) -> ()  [unwired: 8 in, 2 out]
        n120 = Merge Errors(w366, w356) -> (w369:errorcluster)
      }
      frame "Fixed cursor" {
        # "Duplicate this frame when creating new messages.  Change this comment in the duplicated frame to describe this message."
        n121 = Merge Errors(w375) -> (w374:errorcluster)
      }
      frame "Free cursor" {
        # "Duplicate this frame when creating new messages.  Change this comment in the duplicated frame to describe this message."
        n122 = Merge Errors(w380) -> (w379:errorcluster)
      }
      frame Default {
        # "'Default' case only runs if there is a message that isn't defined in any of the other cases.  Output a programming error."
        n123 = xnode "Error Ring"("parameter 0"=w382) -> ("error out"=w381:errorcluster)
      }
    }
    n124 = call "Error Handler - Message Handling Loop.vi"("error in (no error)"=w88, "Message Queue"=w87) -> ("dup error in"=w89:errorcluster)  [unwired: 8 in, 1 out]
  }
  n125 = while "Data Display Loop" {
    tunnel: w4 -> [w398]
    shift-right: [w393] -> _
    shift-left: FALSE -> [w394]
    stop <- w395 stop-if-true
    # "Data Display Loop"
    n126 = Wait on Notification(notifier=w398) -> (notification=w396:T6, error out=w395:errorcluster)  [unwired: 3 in, 2 out]
    n127 = Unbundle By Name(w396) -> ("Content type"=w397:enum16{"None", "Telemetria", "GPS"})
    n128 = case shown="\"GPS\"" w397 {
      tunnel: w396 -> [_ w406 w476]
      tunnel: w395 -> [_ _ w480]
      tunnel: w394 -> [w399 w403 w474]
      tunnel: [w399 w402 w473] -> w393
      frame "None", Default {
        n129 = local read "Messages with wrong length"() -> (w401:u32)
        n130 = Increment(x=w401) -> (x+1=w400:u32)
        n131 = local write "Messages with wrong length"(w400) -> ()
      }
      frame "Telemetria" {
        n132 = call "Decode data format.vi"("Generic packet"=w406) -> ("XAM Data Packet"=w405:T15, "IDRA Data Packet"=w407:T16, "Telemetria.Data format"=w404:enum16{"IDRA data", "XAM data"})  [unwired: 8 in]
        n133 = Not(x=w403) -> (.not. x?=w402:bool)
        n134 = case shown="\"IDRA data\", Default" w404 {
          tunnel: w407 -> [w409 _]
          tunnel: w405 -> [_ w472]
          frame "IDRA data", Default {
            n135 = Unbundle By Name(w409) -> ("Minutes"=w410:u16, "Seconds/100"=w411:u16, "Voltage"=w417:sgl, "Current"=w420:sgl, "Speed"=w419:sgl, "Temperature 1"=→"Temperature1_top" →"Temperature 1":sgl, "Temperature 2"=→"Temperature2_top" →"Temperature 2":sgl, "Temperature 3"=→"Temperature3_top" →"Temperature 3":sgl, "Humidity 1"=→"Humidity1_top" →"Humidity 1":sgl, "Humidity 2"=→"Humidity2_top" →"Humidity 2":sgl, "Strategy"=→"Strategy_top":u8, "Electric Motor"=→"ElettricMotor_top":bool, "Electronics"=→"Electronics_top":bool, "Emergency"=→"Emergency_top":bool)
            "Voltage_top" <- w417
            "Current_top" <- w420
            "Speed_top" <- w419
            "Speed" <- w419
            "Voltage" <- w417
            "Current" <- w420
            n136 = Divide(x=w411, y=sgl 100.0 ("ID trasmitter")) -> (x/y=w416:sgl)
            n137 = Multiply(x=w410, y=sgl 60.0 ("ID trasmitter")) -> (x*y=w415:sgl)
            n138 = Add(x=w415, y=w416) -> (x+y=w412:sgl)
            n139 = Bundle By Name(cluster=T14 {"Time"=0.0, "Voltage"=0.0, "Current"=0.0, " Speed"=0.0, "ID trasmitter"=0} ("Value In"), "Time"=w412, "Voltage"=w417, "Current"=w420, "Speed"=w419, "ID trasmitter"=0) -> (w421:T14)
            n140 = Quotient & Remainder(x=w411, y=u16 100) -> (x-y*floor(x/y)=w429:u16, floor(x/y)=w430:u16)
            n141 = call "Chart_to_GraphXY_3.vi"("Function"=Chart_to_Graph_enum."AddValue", "Time window"=100, "Value In"=w421) -> ("XY Graph Speed"=→"Speed_Graph":cluster{"Tempi":dbl[], "Valori":dbl[]}[], "XY Graph Current"=→"Current_Graph":cluster{"Tempi":dbl[], "Valori":dbl[]}[], "XY Graph Voltage"=→"Voltage_Graph":cluster{"Tempi":dbl[], "Valori":dbl[]}[])  [unwired: 5 in, 1 out]
            n142 = Format Into String(format string="%d:%d,%d", w410, w430, w429) -> (resulting string=→"TimeRT" →"TimeM":string)  [unwired: 2 in, 1 out]
          }
          frame "XAM data" {
            n143 = Unbundle By Name(w472) -> ("Minutes"=w452:u16, "Seconds/100"=w453:u16, "Supercap Voltage"=w450:sgl, "Battery Voltage"=→"Battery voltage" →"Battery_voltage_top":sgl, "Supercap Current"=w449:sgl, "Speed"=w451:sgl, "EM Temperature"=w471:sgl, "ECU Temperature"=w470:sgl, "ICE Temperature"=w469:sgl, "RPM EM"=→"Electric Motor RPM" →"EM_RPM_top":u16, "RPM ICE"=→"ICE RPM" →"ICE_RPM_top":u16, "Cruise Control"=w448:bool, "Emergency"=w447:bool)
            n144 = local write "Electronics_top"(w448) -> ()
            n145 = local write "Emergency_top"(w447) -> ()
            n146 = local write "Temperature 1"(w471) -> ()
            n147 = local write "Temperature1_top"(w471) -> ()
            n148 = local write "Temperature 2"(w470) -> ()
            n149 = local write "Temperature2_top"(w470) -> ()
            n150 = local write "Temperature 3"(w469) -> ()
            n151 = local write "Temperature3_top"(w469) -> ()
            n152 = Divide(x=w453, y=sgl 100.0 ("ID trasmitter")) -> (x/y=w459:sgl)
            n153 = local write "Speed"(w451) -> ()
            n154 = local write "Speed_top"(w451) -> ()
            n155 = local write "Current"(w449) -> ()
            n156 = local write "Current_top"(w449) -> ()
            n157 = local write "Voltage"(w450) -> ()
            n158 = local write "Voltage_top"(w450) -> ()
            n159 = Multiply(x=w452, y=sgl 60.0 ("ID trasmitter")) -> (x*y=w460:sgl)
            n160 = Add(x=w460, y=w459) -> (x+y=w463:sgl)
            n161 = Bundle By Name(cluster=T14 {"Time"=0.0, "Voltage"=0.0, "Current"=0.0, " Speed"=0.0, "ID trasmitter"=0} ("Value In"), "Time"=w463, "Voltage"=w450, "Current"=w449, "Speed"=w451, "ID trasmitter"=0) -> (w457:T14)
            n162 = Quotient & Remainder(x=w453, y=u16 100) -> (x-y*floor(x/y)=w466:u16, floor(x/y)=w467:u16)
            n163 = Format Into String(format string="%d:%d,%d", w452, w467, w466) -> (resulting string=w464:string)  [unwired: 2 in, 1 out]
            n164 = call "Chart_to_GraphXY_3.vi"("Function"=Chart_to_Graph_enum."AddValue", "Time window"=100, "Value In"=w457) -> ("XY Graph Speed"=w441:cluster{"Tempi":dbl[], "Valori":dbl[]}[], "XY Graph Current"=w442:cluster{"Tempi":dbl[], "Valori":dbl[]}[], "XY Graph Voltage"=w443:cluster{"Tempi":dbl[], "Valori":dbl[]}[])  [unwired: 5 in, 1 out]
            n165 = local write "TimeRT"(w464) -> ()
            n166 = local write "Voltage_Graph"(w443) -> ()
            n167 = local write "Current_Graph"(w442) -> ()
            n168 = local write "Speed_Graph"(w441) -> ()
          }
        }
      }
      frame "GPS" {
        w477 = Gps_Map_Graph_enum."SetValue" ("Function")
        n169 = Not(x=w474) -> (.not. x?=w473:bool)
        n170 = Unbundle By Name(w476) -> ("GPS"=w475:T7)
        n171 = control-ref of="Mini Map"() -> (w479:refnum<vi>)
        n172 = control-ref of="Map"() -> (w478:refnum<vi>)
        n173 = call "GPS Map Graph.vi"("Error In"=w480, "Function"=w477, "Coordinates"=w475, "Map ref in"=w478) -> ()  [unwired: 6 in, 2 out]
        n174 = call "GPS Map Graph.vi"("Error In"=w480, "Function"=w477, "Coordinates"=w475, "Map ref in"=w479) -> ()  [unwired: 6 in, 2 out]
      }
    }
    "RX" <- w394
  }
  n175 = call "Acquisition Message Loop.vi"("error in (no error)"=w15, "Data Queue"=w8, "Data Notifier"=w4, "Message Queues"=w17) -> ("error out"=w19:errorcluster)  [unwired: 7 in]
  n176 = call "Logging Message Loop.vi"("error in (no error)"=w15, "Data Queue"=w8, "Message Queues"=w17) -> ("error out"=w16:errorcluster)  [unwired: 8 in]
  n177 = Unregister For Events(event registration refnum=w13, error in=w22) -> (error out=w14:errorcluster)
  n178 = Merge Errors(w14, w23, w19, w16) -> (w5:errorcluster)
  n179 = call "Destroy User Event - Stop.vi"("error in (no error)"=w5, "User Event - Stop"=w20) -> ("error out"=w7:errorcluster)  [unwired: 9 in]
  n180 = disable-structure shown="Default" {
    disable-tunnel: w7 -> [_ _]
    frame condition #0 (active) {
    }
    frame condition #1 {
      # "Call Quit LabVIEW if running as a built application."
      n181 = Quit LabVIEW() -> ()  [unwired: 1 in]
    }
  }
